vi "Engine - Initialize HW.vi"(8 "error in (no error)":errorcluster, 10 "DMM-Switch Configuration":T1 {"DMM Resolution in Digits" items=["3 1/2"=3.5, "4 1/2"=4.5, "5 1/2"=5.5, "6 1/2"=6.5, "7 1/2"=7.5]}) -> (0 "error out":errorcluster, 2 "DMM Ref Out":refnum<k15>, 3 "Switch Ref Out":refnum<k15>)   [LabVIEW 2015, in "DMM-SWITCH-ScanList Engine.lvlib"]
doc: "Initialize and configure Switch and DMM devices for a Hardware Triggered Scan List Measurement configured with the parameters coming from the DMM-Switch Configuration Cluster."
uses:
  DMM-SWITCH-ScanList Engine.lvlib
  TypeDefs/DMM-Switch Configuration.ctl
  <instrlib>/niDMM/nidmm.llb/niDMM Function.ctl
  <instrlib>/niDMM/nidmm.llb/niDMM Resolution in Digits.ctl
  <instrlib>/niSwitch/niSwitch.LLB/niSwitch Topologies.ctl
  <instrlib>/niSwitch/niSwitch.LLB/niSwitch Trigger Input.ctl
  <instrlib>/niSwitch/niSwitch.LLB/niSwitch Scan Advanced Output.ctl
  <instrlib>/niDMM/nidmm.llb/niDMM Measurement Complete.ctl
  <instrlib>/niDMM/nidmm.llb/niDMM Trigger.ctl
  <instrlib>/niDMM/nidmm.llb/niDMM Sample Trigger.ctl
  <instrlib>/niDMM/nidmm.llb/niDMM Configure Measurement Digits.vi
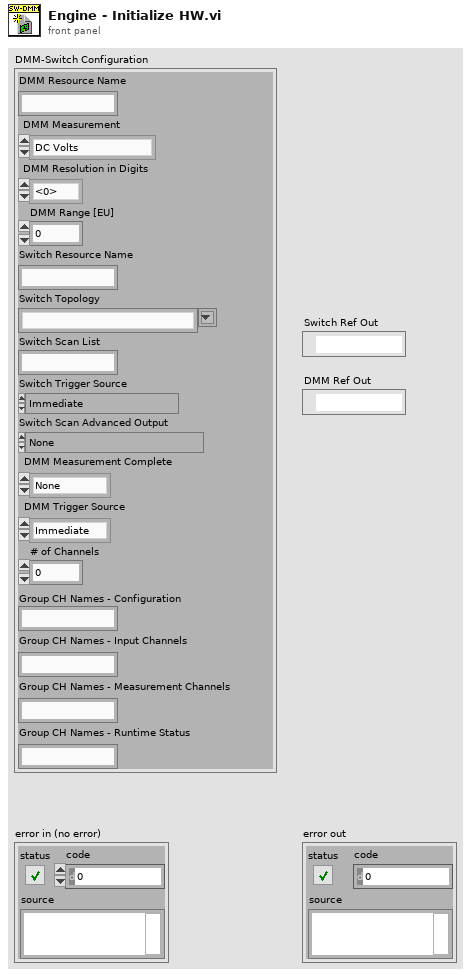
[diagram p1: front panel]
types:
  T1 = typedef "DMM-SWITCH-ScanList Engine.lvlib/DMM-Switch Configuration.ctl" = cluster{"DMM Resource Name":string, "DMM Measurement":T2, "DMM Resolution in Digits":T3, "DMM Range [EU]":dbl, "Switch Resource Name":string, "Switch Topology":T4, "Switch Scan List":string, "Switch Trigger Source":T5, "Switch Scan Advanced Output":T6, "DMM Measurement Complete":T7, "DMM Trigger Source":T8, "# of Channels":u32, "Group CH Names - Configuration":string, "Group CH Names - Input Channels":string, "Group CH Names - Measurement Channels":string, "Group CH Names - Runtime Status":string}
  T2 = typedef "niDMM Function.ctl" = enum16{"DC Volts", "AC Volts", "DC Current", "AC Current", "2-wire Resistance", "4-wire Resistance", "Diode", "Frequency", "Period", "AC Volts DC Coupled", "Capacitance", "Inductance", "Temperature"}
  T3 = typedef "niDMM Resolution in Digits.ctl" = dbl
  T4 = typedef "niSwitch Topologies.ctl" = string
  T5 = typedef "niSwitch Trigger Input.ctl" = enum16{"Immediate", "External", "TTL0", "TTL1", "TTL2", "TTL3", "TTL4", "TTL5", "TTL6", "TTL7", "ECL0", "ECL1", "PXI Star", "Software Trigger Function", "Rear Connector", "Front Connector", "Rear Connector of Module 1", "Rear Connector of Module 2", "Rear Connector of Module 3", "Rear Connector of Module 4", "Rear Connector of Module 5", "Rear Connector of Module 6", "Rear Connector of Module 7", "Rear Connector of Module 8", "Rear Connector of Module 9", "Rear Connector of Module 10", "Rear Connector of Module 11", "Rear Connector of Module 12", "Front Connector of Module 1", "Front Connector of Module 2", "Front Connector of Module 3", "Front Connector of Module 4", "Front Connector of Module 5", "Front Connector of Module 6", "Front Connector of Module 7", "Front Connector of Module 8", "Front Connector of Module 9", "Front Connector of Module 10", "Front Connector of Module 11", "Front Connector of Module 12"}
  T6 = typedef "niSwitch Scan Advanced Output.ctl" = enum16{"None", "External", "TTL0", "TTL1", "TTL2", "TTL3", "TTL4", "TTL5", "TTL6", "TTL7", "ECL0", "ECL1", "PXI Star", "Rear Connector", "Front Connector", "Rear Connector Module 1", "Rear Connector Module 2", "Rear Connector Module 3", "Rear Connector Module 4", "Rear Connector Module 5", "Rear Connector Module 6", "Rear Connector Module 7", "Rear Connector Module 8", "Rear Connector Module 9", "Rear Connector Module 10", "Rear Connector Module 11", "Rear Connector Module 12", "Front Connector Module 1", "Front Connector Module 2", "Front Connector Module 3", "Front Connector Module 4", "Front Connector Module 5", "Front Connector Module 6", "Front Connector Module 7", "Front Connector Module 8", "Front Connector Module 9", "Front Connector Module 10", "Front Connector Module 11", "Front Connector Module 12"}
  T7 = typedef "niDMM Measurement Complete.ctl" = enum16{"None", "External", "TTL 0", "TTL 1", "TTL 2", "TTL 3", "TTL 4", "TTL 5", "TTL 6", "TTL 7", "LBR Trig 0"}
  T8 = typedef "niDMM Trigger.ctl" = enum16{"Immediate", "External", "TTL 0", "TTL 1", "TTL 2", "TTL 3", "TTL 4", "TTL 5", "TTL 6", "Software", "TTL 7", "PXI Star", "LBR Trig 1", "Aux Trig 1"}
  T9 = typedef "niDMM Sample Trigger.ctl" = enum16{"Immediate", "External", "TTL 0", "TTL 1", "TTL 2", "TTL 3", "TTL 4", "TTL 5", "TTL 6", "Interval", "Software", "TTL 7", "PXI Star", "LBR Trig 1", "Aux Trig 1"}
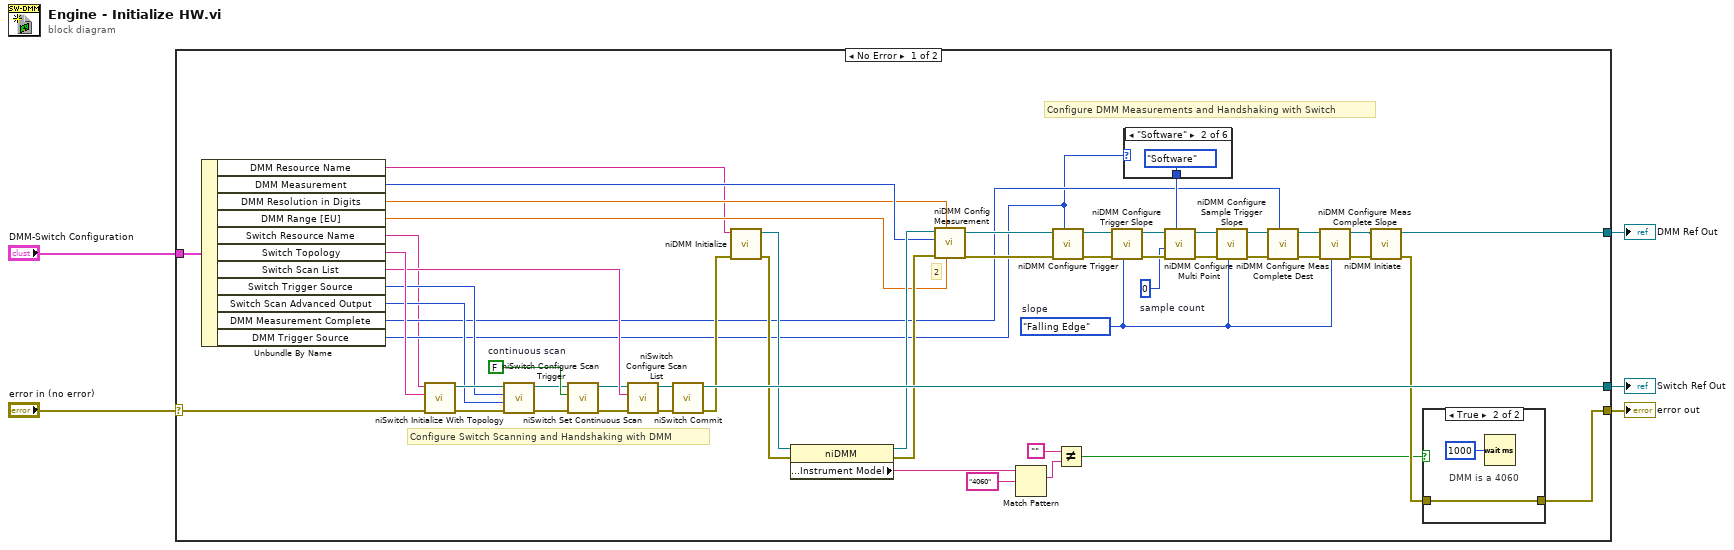
[diagram p0: block diagram]
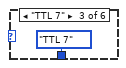
[diagram p4: hidden frame]
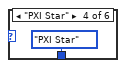
[diagram p5: hidden frame]
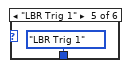
[diagram p6: hidden frame]
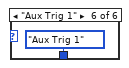
[diagram p7: hidden frame]
diagram:
  n1 = case shown="No Error" "error in (no error)" {
    selector: "error in (no error)" -> [w19 w68]
    tunnel: [w58 _] -> w5
    tunnel: [w57 w68] -> w4
    tunnel: [w56 _] -> w3
    tunnel: "DMM-Switch Configuration" -> [w26 _]
    frame No Error {
      w36 = enum16{"Rising Edge", "Falling Edge"}."Falling Edge"  # slope
      w47 = 0  # sample count
      w27 = FALSE  # continuous scan
      # "Configure DMM Measurements and Handshaking with Switch"
      # "Configure Switch Scanning and Handshaking with DMM"
      # "2"
      n2 = Unbundle By Name(w26) -> ("DMM Resource Name"=w8:string, "DMM Measurement"=w15:T2, "DMM Resolution in Digits"=w14:T3, "DMM Range [EU]"=w13:dbl, "Switch Resource Name"=w6:string, "Switch Topology"=w30:T4, "Switch Scan List"=w28:string, "Switch Trigger Source"=w12:T5, "Switch Scan Advanced Output"=w11:T6, "DMM Measurement Complete"=w10:T7, "DMM Trigger Source"=w9:T8)
      n3 = call <instrlib>:"niSwitch Initialize With Topology.vi"("error in (no error)"=w19, "topology name"=w30, "resource name"=w6) -> ("error out"=w7:errorcluster, "instrument handle out"=w24:refnum<k15>)  [unwired: 2 in, 5 out]
      n4 = call <instrlib>:"niSwitch Configure Scan Trigger.vi"("error in (no error)"=w7, "scan advanced output (External)"=w11, "trigger input (External)"=w12, "instrument handle"=w24) -> ("error out"=w29:errorcluster, "instrument handle out"=w25:refnum<k15>)  [unwired: 1 in, 5 out]
      n5 = call <instrlib>:"niSwitch Set Continuous Scan.vi"("error in (no error)"=w29, "continuous scan (False)"=w27, "instrument handle"=w25) -> ("error out"=w18:errorcluster, "instrument handle out"=w23:refnum<k15>)  [unwired: 7 out]
      n6 = call <instrlib>:"niSwitch Configure Scan List.vi"("error in (no error)"=w18, "scan list"=w28, "instrument handle"=w23) -> ("error out"=w17:errorcluster, "instrument handle out"=w22:refnum<k15>)  [unwired: 1 in, 6 out]
      n7 = call <instrlib>:"niSwitch Commit.vi"("error in (no error)"=w17, "instrument handle"=w22) -> ("error out"=w16:errorcluster, "instrument handle out"=w58:refnum<k15>)  [unwired: 8 out]
      n8 = call <instrlib>:"niDMM Initialize.vi"("error in (no error)"=w16, "Instrument Descriptor"=w8) -> ("error out"=w20:errorcluster, "instrument handle out"=w34:refnum<k15>)  [unwired: 2 in, 6 out]
      n9 = property class="niDMM"(reference=w34, error in=w20) -> (reference out=w33:refnum<k15>, error out=w21:errorcluster, "Inherent IVI Attributes:Instrument Identification:Instrument Model"=w35:string)
      n10 = call-poly <instrlib>:"niDMM Config Measurement.vi"("Range"=w13, "Resolution in Digits"=w14, "error in (no error)"=w21, "Function"=w15, "instrument handle"=w33) -> ("error out"=w31:errorcluster, "instrument handle out"=w32:refnum<k15>)  [unwired: 5 out]
      n11 = Match Pattern(string=w35, regular expression="4060") -> (match substring=w44:string)  [unwired: 4 out]
      n12 = call <instrlib>:"niDMM Configure Trigger.vi"("Trigger Source"=w9, "error in (no error)"=w31, "instrument handle"=w32) -> ("error out"=w52:errorcluster, "instrument handle out"=w53:refnum<k15>)  [unwired: 1 in, 6 out]
      n13 = Not Equal?(x="", y=w44) -> (x != y?=w54:bool)
      n14 = call <instrlib>:"niDMM Configure Trigger Slope.vi"("Slope"=w36, "error in (no error)"=w52, "instrument handle"=w53) -> ("error out"=w50:errorcluster, "instrument handle out"=w51:refnum<k15>)  [unwired: 7 out]
      n15 = case shown="\"Software\"" w9 {
        selector: w9 -> [w62 _ _ _ _ _]
        tunnel: [w62 niDMM_Sample_Trigger."Software" ("Sample Trigger") niDMM_Sample_Trigger."TTL 7" ("Sample Trigger") niDMM_Sample_Trigger."PXI Star" ("Sample Trigger") niDMM_Sample_Trigger."LBR Trig 1" ("Sample Trigger") niDMM_Sample_Trigger."Aux Trig 1" ("Sample Trigger")] -> w46
        frame "Immediate", Default {
        }
        frame "Software" {
        }
        frame "TTL 7" {
        }
        frame "PXI Star" {
        }
        frame "LBR Trig 1" {
        }
        frame "Aux Trig 1" {
        }
      }
      n16 = call <instrlib>:"niDMM Configure Multi Point.vi"("Sample Trigger"=w46, "error in (no error)"=w50, "Sample Count"=w47, "instrument handle"=w51) -> ("error out"=w48:errorcluster, "instrument handle out"=w49:refnum<k15>)  [unwired: 2 in, 4 out]
      n17 = call <instrlib>:"niDMM Configure Sample Trigger Slope.vi"("Slope"=w36, "error in (no error)"=w48, "instrument handle"=w49) -> ("error out"=w42:errorcluster, "instrument handle out"=w41:refnum<k15>)  [unwired: 7 out]
      n18 = call <instrlib>:"niDMM Configure Meas Complete Dest.vi"("Measurement Complete Destination"=w10, "error in (no error)"=w42, "instrument handle"=w41) -> ("error out"=w37:errorcluster, "instrument handle out"=w40:refnum<k15>)  [unwired: 7 out]
      n19 = call <instrlib>:"niDMM Configure Meas Complete Slope.vi"("Slope"=w36, "error in (no error)"=w37, "instrument handle"=w40) -> ("error out"=w38:errorcluster, "instrument handle out"=w39:refnum<k15>)  [unwired: 7 out]
      n20 = call <instrlib>:"niDMM Initiate.vi"("error in (no error)"=w38, "instrument handle"=w39) -> ("error out"=w55:errorcluster, "instrument handle out"=w56:refnum<k15>)  [unwired: 8 out]
      n21 = case shown="True" w54 {
        tunnel: w55 -> [w59 w60]
        tunnel: [w59 w60] -> w57
        frame False {
          # "DMM is \nnot a 4060"
        }
        frame True {
          # "DMM is a 4060"
          n22 = Wait (ms)(milliseconds to wait=u32 1000 ("millisecond multiple")) -> ()  [unwired: 1 out]
        }
      }
    }
    frame Error {
    }
  }
  "Switch Ref Out" <- w5
  "error out" <- w4
  "DMM Ref Out" <- w3
